vi "Send.vi"(10 "Error":errorcluster) -> (3 "Set Error Msg out":refnum<class "Set Error Msg.lvclass">)   [LabVIEW 2021, in "Set Error.lvlib" / "Set Error Msg.lvclass"]
uses:
  Set Error Msg.lvclass
  Set Error Msg.lvclass/Set Error Msg.ctl
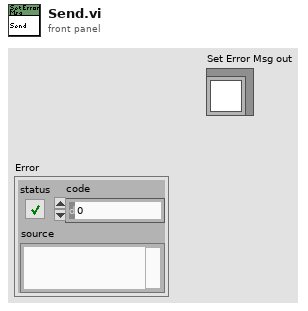
[diagram p1: front panel]
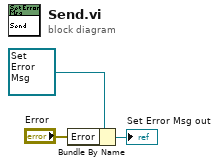
[diagram p0: block diagram]
diagram:
  n1 = Bundle By Name(cluster=refnum<class "Set Error Msg.lvclass"> refnum ("Error Msg Strategy out"), "Error"="Error") -> (→"Set Error Msg out":refnum<class "Set Error Msg.lvclass">)
